vi "kuirs_事件_生产者消费者_多图像获取 1.vi"() -> ()   [LabVIEW 2019]
doc: "该模板用于创建生产者／消费者模式的应用程序，以事件驱动的方式，生成队列中的项。如需通过响应事件实现代码的异步执行，同时不影响用户界面的响应速度，可考虑用该模式替代“用户界面事件处理器”模式。"
uses:
  <vilib>/userdefined/High Color/IMAQdx.ctl
  <vilib>/vision/driver/NI_Vision_Acquisition_Software.lvlib
  <vilib>/vision/NI_Vision_Development_Module.lvlib
panel:
  out "Image":T1(plugin-control)
  out "Images":T1(plugin-control)
  in  "SNAP":bool caption="元素入队列"
  in  "STOP":bool caption="停止"
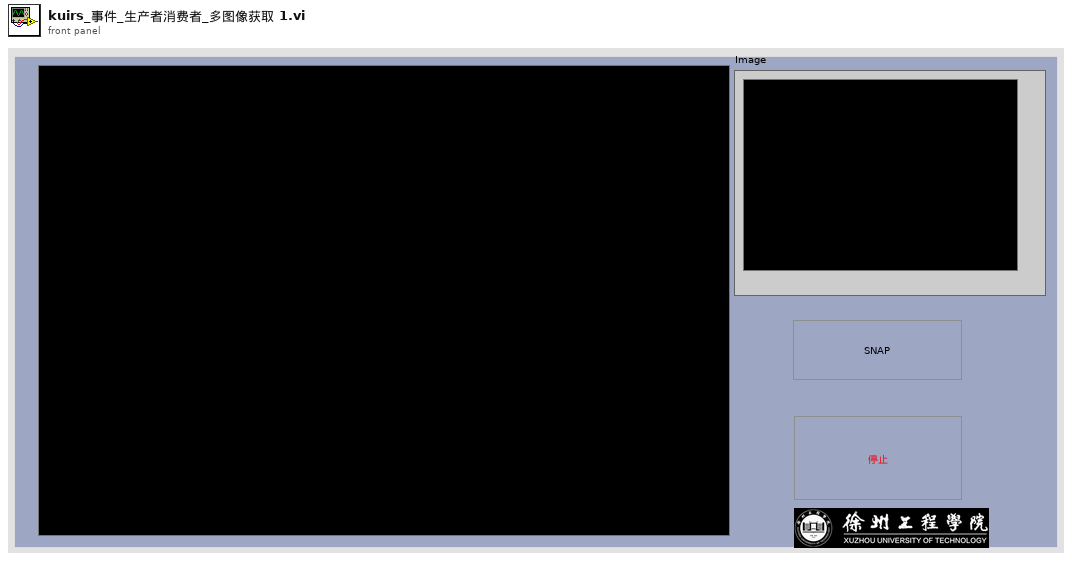
[diagram p1: front panel]
types:
  T1 = typedef "IMAQ Image.ctl" = refnum<image>
  T2 = typedef "Image Type" = u32
  T3 = cluster{"Browser Size":cluster{"X":i32, "Y":i32}, "Images per Line":i32, "Background Color":u32, "Frame Size":i32, "Frame Style":enum16{"Raised", "Bevelled", "Outline", "Hidden", "Step", "Raised Outline"}}
  T4 = typedef "IMAQdx.ctl" = refnum<k21>
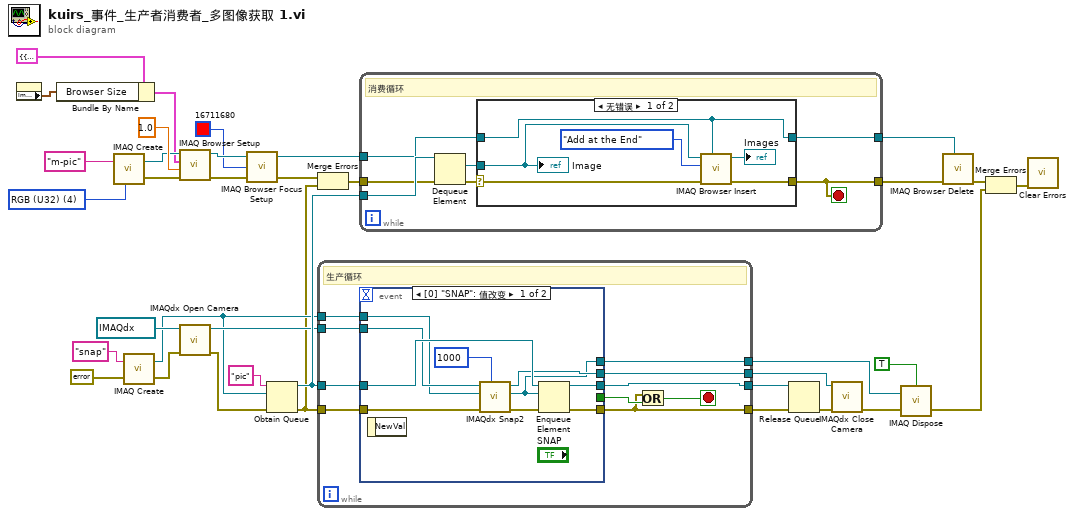
[diagram p0: block diagram]
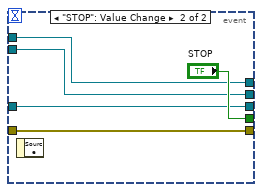
[diagram p3: hidden frame]
diagram:
  w7 = T2 4 items=["Grayscale (U8)", "Grayscale (I16)", "Grayscale (SGL)", "Complex (CSG)", "RGB (U32)", "HSL (U32)", "RGB (U64)", "Grayscale (U16)"] ("Image Type")
  n1 = property on="Images" class="ImageControl"() -> ("Image Area Size"=w9:cluster{"Width":u32, "Height":u32})  [unwired: 2 in, 2 out]
  n2 = Bundle By Name(cluster=T3 {"Browser Size"={"X"=640, "Y"=480}, "Images per Line"=6, "Background Color"=11053224, "Frame Size"=1, "Frame Style"=enum."Raised"} ("Browser Info"), "Browser Size"=w9) -> (w8:T3)
  n3 = call "IMAQ Create"("Image Name"="m-pic", "Image Type"=w7) -> ("New Image"=w19:T1, "error out"=w6:errorcluster)  [unwired: 3 in]
  n4 = call "IMAQ Create"("Image Name"="snap", "error in (no error)"=errorcluster {"status"=FALSE, "code"=0, "source"=""}) -> ("New Image"=w24:T1, "error out"=w33:errorcluster)  [unwired: 3 in]
  n5 = call "IMAQ Browser Setup"("error in (no error)"=w6, "Image Ratio"=sgl 1.0, "Browser Info"=w8, "Image In"=w19) -> ("error out"=w5:errorcluster, "Image Browser Out"=w13:T1)  [unwired: 2 out]
  n6 = call <vilib>:"IMAQdx Open Camera.vi"("error in"=w33, "Session In"=T4 "cam1") -> ("error out"=w23:errorcluster, "Session Out"=w31:T4)  [unwired: 8 in]
  n7 = call "IMAQ Browser Focus Setup"("error in (no error)"=w5, "Focus Color"=u32 16711680, "Image Browser In"=w13) -> ("error out"=w4:errorcluster, "Image Browser Out"=w12:T1)  [unwired: 1 in]
  n8 = Obtain Queue(name (unnamed)="pic" ("名称（未命名）"), element data type=w24, error in (no error)=w23) -> (queue out=w35:refnum<queue>, error out=w3:errorcluster)  [unwired: 2 in, 1 out]
  n9 = Merge Errors(w4, w3) -> (w2:errorcluster)
  n10 = while {
    tunnel: w35 -> [w46]
    tunnel: w31 -> [w41]
    tunnel: w24 -> [w40]
    tunnel: [w39] -> w30
    tunnel: [w38] -> w28
    tunnel: w3 -> [w45]
    tunnel: [w42] -> w36
    tunnel: [w37] -> w25
    stop <- w43 stop-if-true
    # "生产循环"
    n11 = event shown="[0] \"SNAP\": 值改变" {
      selector: _ -> [_ _]
      dyn-events: _ -> [_ _]
      timeout: _ -> [_ _]
      tunnel: w46 -> [w56 w59]
      tunnel: w45 -> [w49 w60]
      tunnel: [w55 w60] -> w42
      tunnel: [_ "STOP"] -> w44
      tunnel: w41 -> [w54 w58]
      tunnel: w40 -> [w53 w57]
      tunnel: [w51 w57] -> w38
      tunnel: [w52 w58] -> w39
      tunnel: [w50 w59] -> w37
      event "SNAP": Value Change {
        n12 = event-data() -> ()  [unwired: 1 in, 1 out]
        n13 = call <vilib>:"IMAQdx Snap2.vi"("Timeout (ms)"=1000, "error in"=w49, "Image In"=w53, "Session In"=w54) -> ("error out"=w47:errorcluster, "Image Out"=w51:T1, "Session Out"=w52:T4)  [unwired: 5 in]
        n14 = Enqueue Element(queue=w56, element=w51, error in (no error)=w47) -> (queue out=w50:refnum<queue>, error out=w55:errorcluster)  [unwired: 1 in, 1 out]
      }
      event "STOP": Value Change {
        n15 = event-data() -> ()  [unwired: 1 in, 1 out]
      }
    }
    n16 = Or(x=w42, y=w44) -> (x .or. y?=w43:bool)
  }
  n17 = while {
    tunnel: w35 -> [w68]
    tunnel: w12 -> [w65]
    tunnel: [w64] -> w17
    tunnel: [w63] -> w16
    tunnel: w2 -> [w62]
    stop <- w63 stop-if-true
    # "消费循环"
    n18 = Dequeue Element(queue=w68, error in (no error)=w62) -> (element=w66:T1, error out=w67:errorcluster)  [unwired: 1 in, 2 out]
    n19 = case shown="无错误" w67 {
      selector: w67 -> [w72 w76]
      tunnel: w66 -> [w69 _]
      tunnel: [w71 w76] -> w63
      tunnel: w65 -> [w70 w75]
      tunnel: [w70 w75] -> w64
      frame No Error {
        n20 = call "IMAQ Browser Insert"("Image Browser In"=w70, "error in (no error)"=w72, "Insertion Mode"=enum16{"Add at First Free", "Add at the End"}."Add at the End", "Image to Add"=w69) -> ("error out"=w71:errorcluster, "Image Browser Out"=→"Images":T1)  [unwired: 3 in, 3 out]
        "Image" <- w69
      }
      frame Error {
      }
    }
  }
  n21 = Release Queue(queue=w25, error in (no error)=w36) -> (error out=w26:errorcluster)  [unwired: 1 in, 2 out]
  n22 = call <vilib>:"IMAQdx Close Camera.vi"("error in"=w26, "Session In"=w30) -> ("error out"=w29:errorcluster)  [unwired: 9 in]
  n23 = call "IMAQ Dispose"("All Images? (No)"=TRUE, "Image"=w28, "error in (no error)"=w29) -> ("error out"=w14:errorcluster)  [unwired: 3 in]
  n24 = call "IMAQ Browser Delete"("Image Browser In"=w17, "error in (no error)"=w16) -> ("error out"=w15:errorcluster)  [unwired: 5 in, 4 out]
  n25 = Merge Errors(w15, w14) -> (w1:errorcluster)
  n26 = call <vilib>:"Clear Errors.vi"("error in (no error)"=w1) -> ()  [unwired: 5 in, 2 out]
